vi "Degree_To_Bits_Conversion.vi"(10 "Degree":dbl[](array[numeric])) -> (2 "Bit positions":u16[](array[numeric]))   [LabVIEW 2015]
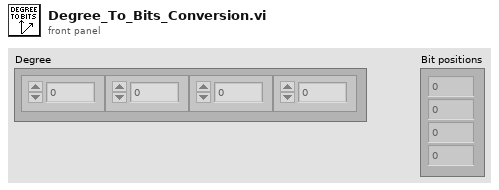
[diagram p1: front panel]
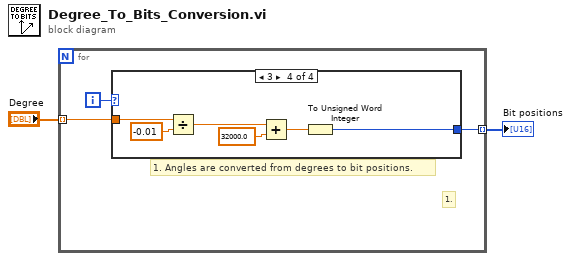
[diagram p0: block diagram]
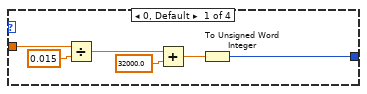
[diagram p2: hidden frame]
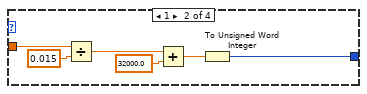
[diagram p3: hidden frame]
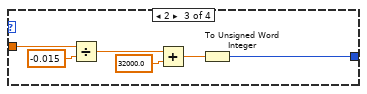
[diagram p4: hidden frame]
diagram:
  n1 = for {
    tunnel: "Degree" -> [w4] mode=indexing
    tunnel: [w3] -> w1 mode=indexing
    i -> [w5]
    # "1."
    # "1. Angles are converted from degrees to bit positions."
    n2 = case shown="3" w5 {
      tunnel: w4 -> [w11 w13 w19 w25]
      tunnel: [w6 w12 w18 w24] -> w3
      frame 0, Default {
        n3 = Divide(x=w11, y=0.015) -> (x/y=w9:dbl)
        n4 = Add(x=w9, y=32000.0) -> (x+y=w7:dbl)
        n5 = To Unsigned Word Integer(number=w7) -> (unsigned 16bit integer=w6:u16)
      }
      frame 1 {
        n6 = Divide(x=w13, y=0.015) -> (x/y=w15:dbl)
        n7 = Add(x=w15, y=32000.0) -> (x+y=w17:dbl)
        n8 = To Unsigned Word Integer(number=w17) -> (unsigned 16bit integer=w12:u16)
      }
      frame 2 {
        n9 = Divide(x=w19, y=-0.015) -> (x/y=w21:dbl)
        n10 = Add(x=w21, y=32000.0) -> (x+y=w23:dbl)
        n11 = To Unsigned Word Integer(number=w23) -> (unsigned 16bit integer=w18:u16)
      }
      frame 3 {
        n12 = Divide(x=w25, y=-0.01) -> (x/y=w27:dbl)
        n13 = Add(x=w27, y=32000.0) -> (x+y=w29:dbl)
        n14 = To Unsigned Word Integer(number=w29) -> (unsigned 16bit integer=w24:u16)
      }
    }
  }
  "Bit positions" <- w1
